vi "ReceiveMessage.vi"(6 "Timeout(100)":i32=100, 8 "error in (no error)":errorcluster, 9 "Priority Action":string, 10 "Default Action":string, 11 "Qbus in":refnum<class "Qbus.lvclass">) -> (0 "error out":errorcluster, 1 "MsgValue":variant, 2 "Action":string, 3 "Qbus out":refnum<class "Qbus.lvclass">, 4 "Exit":bool)   [LabVIEW 2017, in "McsaStartupAnalysis.lvlib"]
uses:
  <vilib>/addons/InsightCM/Devices/Shared/Mcsa/McsaStartupAnalysis/McsaStartupAnalysis.lvlib
  <vilib>/addons/Qbus/Qbus.lvclass
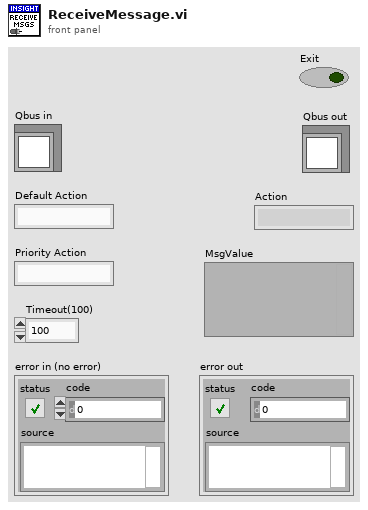
[diagram p1: front panel]
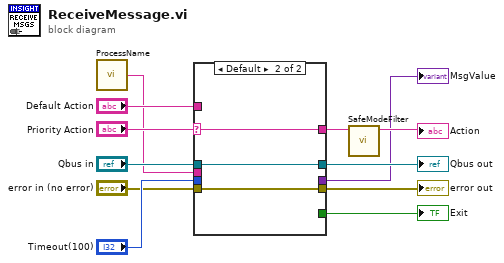
[diagram p0: block diagram]
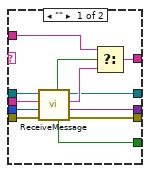
[diagram p2: hidden frame]
diagram:
  n1 = call <vilib>:"ProcessName.vi"() -> ("ProcessName"=w1:string)  [unwired: 5 in]
  n2 = case shown="Default" "Priority Action" {
    selector: "Priority Action" -> [_ w25]
    tunnel: "error in (no error)" -> [w15 w27]
    tunnel: [w21 w27] -> w5
    tunnel: [w20 _] -> w4
    tunnel: [w16 _] -> w2
    tunnel: "Default Action" -> [w24 _]
    tunnel: [w23 w25] -> w11
    tunnel: [w18 w26] -> w10
    tunnel: "Timeout(100)" -> [w14 _]
    tunnel: "Qbus in" -> [w17 w26]
    tunnel: w1 -> [w13 _]
    frame "" {
      n3 = call <vilib>:"ReceiveMessage.vi"("error in (no error)"=w15, "timeout (0)"=w14, "process name"=w13, "Qbus in"=w17) -> ("error in (no error)"=w21:errorcluster, "message value"=w20:variant, "message name"=w19:string, "Qbus out"=w18:refnum<class "Qbus.lvclass">, "exit"=w16:bool, "timed out"=w22:bool)  [unwired: 2 in]
      n4 = Select(t=w24, s=w22, f=w19) -> (s? t:f=w23:string)
    }
    frame Default {
    }
  }
  "Qbus out" <- w10
  "error out" <- w5
  "MsgValue" <- w4
  "Exit" <- w2
  n5 = call <vilib>:"SafeModeFilter.vi"("action in"=w11) -> ("action out"=→"Action":string)  [unwired: 10 in]
